vi "Motor and Two Photon System_Main.vi"() -> ()   [LabVIEW 2016]
doc: "This Continuous Measurement sample project is based on the Queued Message Handler template.\n\nThe Event Handling Loop generates messages based on user interface actions.\n\nThe Message Handling Loop processes messages generated by the Event Handling Loop, or by other messages. There are also Acquisition and Logging message handling loop subVIs, and a chart updating loop."
uses:
  Settings/Settings.ctl
  Acquisition/Hardware Configuration.ctl
  Logging/Logging Configuration.ctl
  Motor Speed/MSpeed AO HW Config.ctl
  Motor Control/Motor Control Config.ctl
  Motor Control/Speed and Duration.ctl
  2P Trigger/2P Trigger Config.ctl
  controls/UI Data.ctl
  controls/UI State.ctl
  support/Message Queue/Enqueue Message (Single).vi
  <vilib>/Utility/error.llb/Error Cluster From Error Code.vi
  <vilib>/ErrorRing/Error Ring.xnode
  Acquisition/Acquisition.lvlib
  Logging/Logging.lvlib
  Settings/Settings.lvlib
  support/User Event - Stop/User Event - Stop.lvlib
  support/Message Queue/Message Queue.lvlib
  Motor Speed/Motor Speed AO.lvlib
  Motor Control/Motor Control.lvlib
  2P Trigger/2P Trigger.lvlib
panel:
  out "Data":waveform(dbl)[](graph)
  in  "Force Trigger":bool
  in  "Settings":bool
  in  "Start":bool
  in  "Stop":bool
  out "Status":string
  in  "Exit":bool
  # "Continuous Measurement and Logging (NI-DAQmx)"
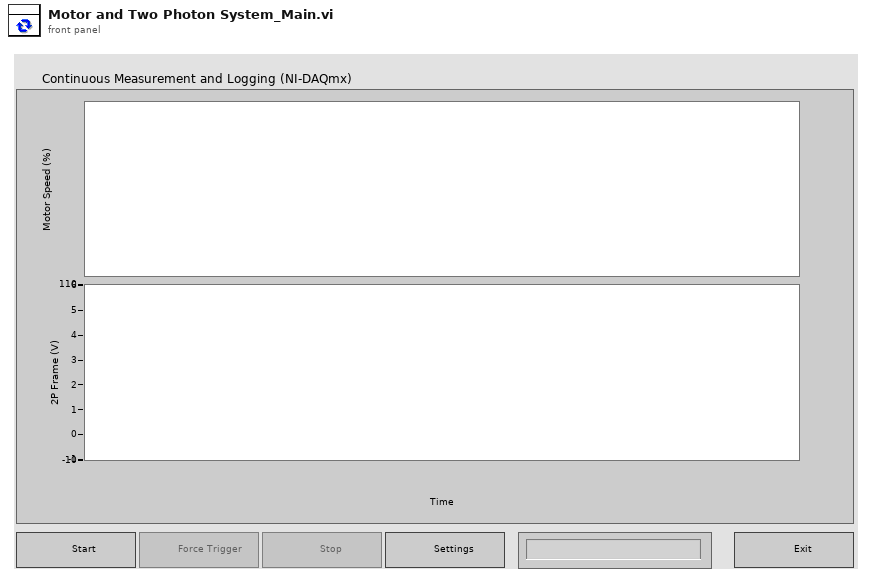
[diagram p1: front panel]
types:
  T1 = typedef "UI State.ctl" = enum16{"Idle", "Acquiring and Logging", "Waiting for Exit", "Waiting for Exit (Acq Stopped)", "Waiting for Exit (Log Stopped)", "Waiting for Stop", "Waiting for Stop (Acq Stopped)", "Waiting for Stop (Log Stopped)"}
  T2 = typedef "UI Data.ctl" = cluster{"Start Ref":refnum<vi>, "Trigger Ref":refnum<vi>, "Stop Ref":refnum<vi>, "Settings Ref":refnum<vi>, "Status Ref":refnum<vi>, "Exit Ref":refnum<vi>, "Data Ref":refnum<vi>}
  T3 = typedef "Settings.lvlib/Settings.ctl" = cluster{"Hardware Configuration":T4, "Logging Configuration":T5, "MSpeed AO HW Config":T6, "Motor Config":T7, "2P Trigger Config":T9}
  T4 = typedef "Acquisition.lvlib/Hardware Configuration.ctl" = cluster{"DAQmx Channel":tag, "Max Input":dbl, "Min Input":dbl, "Sample Rate":dbl, "DAQmx Task":refnum<k21>}
  T5 = typedef "Logging.lvlib/Logging Configuration.ctl" = cluster{"Log File Base Path":path, "TDMS File Reference":refnum<k34>, "Samples to Save":u32, "Trigger - Time":u32, "Trigger - Threshold":dbl, "Trigger - Channel":u32, "Enable Time Trigger":bool, "Enable Threshold Trigger":bool, "Always Log":bool}
  T6 = typedef "Motor Speed AO.lvlib/MSpeed AO HW Config.ctl" = cluster{"MSpeed AO Channel":tag, "Sample Rate(Hz)":dbl, "MSpeed AO Task":refnum<k21>}
  T7 = typedef "Motor Control.lvlib/Motor Control Config.ctl" = cluster{"VISA resource name":refnum<visa-resource-name>, "Speed and Duration":T8[]}
  T8 = typedef "Motor Control.lvlib/Speed and Duration.ctl" = cluster{"Speed (%)":i32, "Duration (sec)":dbl}
  T9 = typedef "2P Trigger.lvlib/2P Trigger Config.ctl" = cluster{"DO Line":tag}
  T10 = typedef "Message Queue.lvlib/All Message Queues.ctl" = cluster{"UI":refnum<queue>, "Acquisition":refnum<queue>, "Logging":refnum<queue>, "Motor Speed":refnum<queue>, "Motor Control":refnum<queue>, "2P Trigger":refnum<queue>}
  T11 = enum8{"Enabled", "Disabled", "Disabled and Grayed Out"}
  T12 = cluster{"MSpeed AO HW Config":T6, "VISA resource name":refnum<visa-resource-name>}
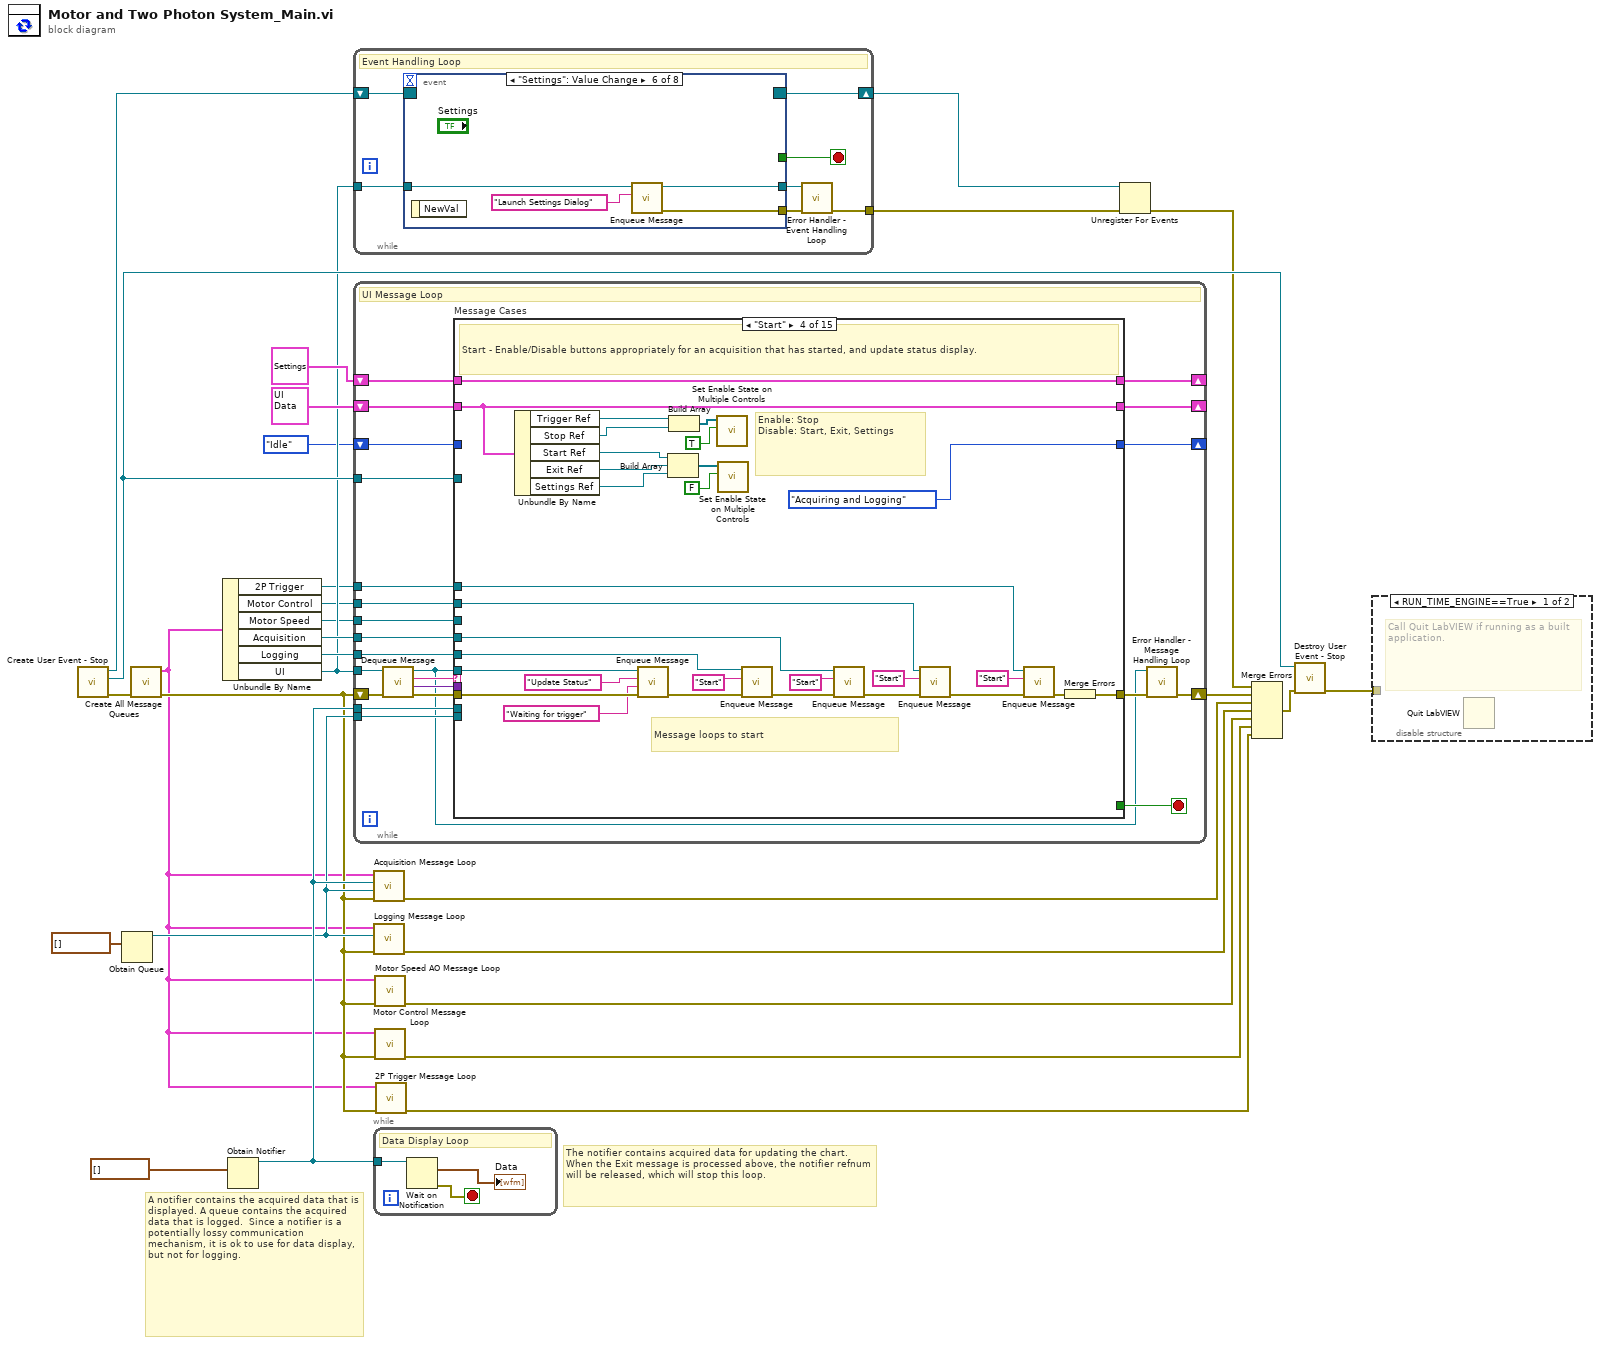
[diagram p0: block diagram]
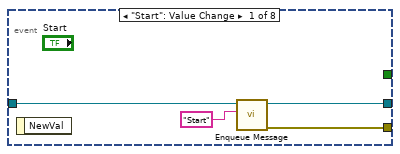
[diagram p3: hidden frame]
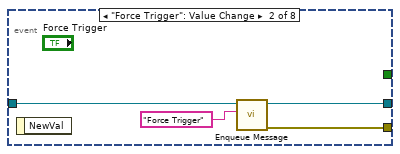
[diagram p4: hidden frame]
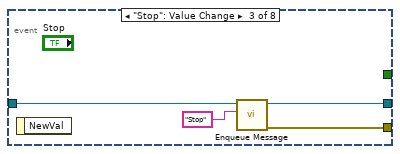
[diagram p5: hidden frame]
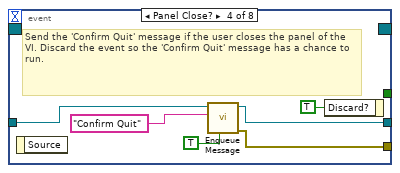
[diagram p6: hidden frame]
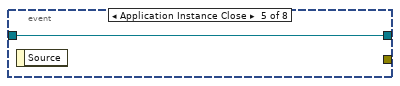
[diagram p7: hidden frame]
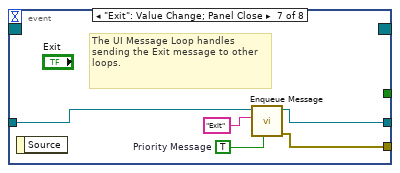
[diagram p8: hidden frame]
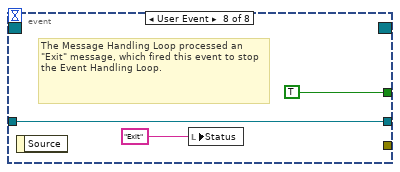
[diagram p9: hidden frame]
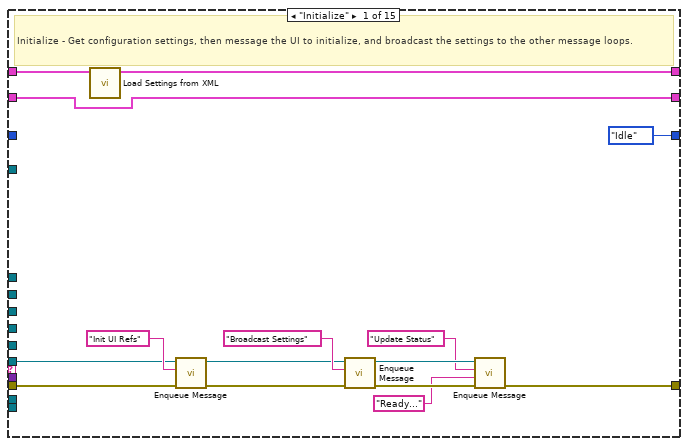
[diagram p10: hidden frame]
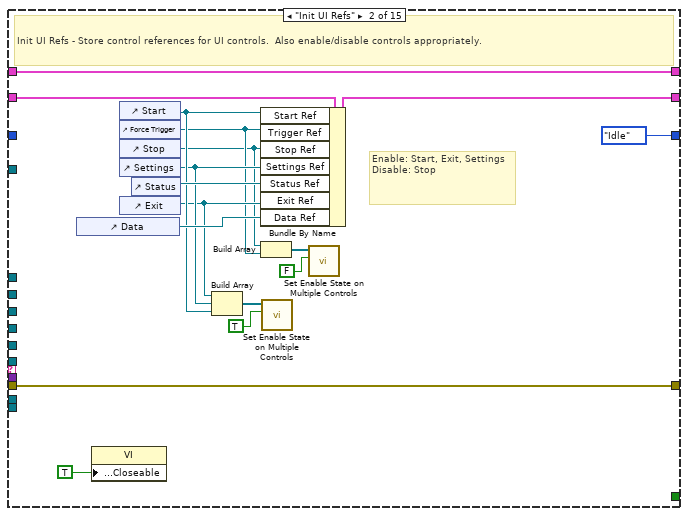
[diagram p11: hidden frame]
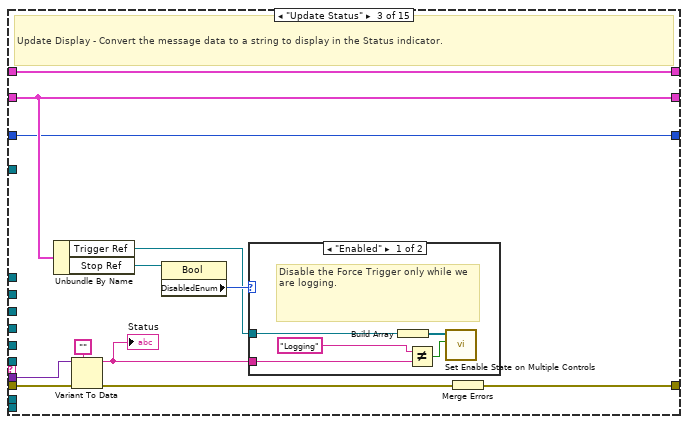
[diagram p12: hidden frame]
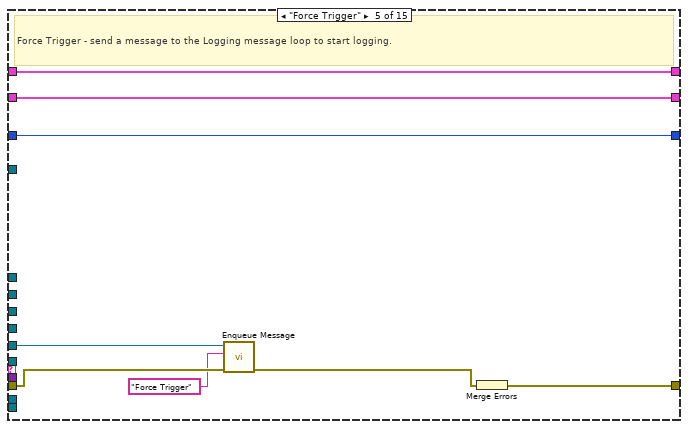
[diagram p14: hidden frame]
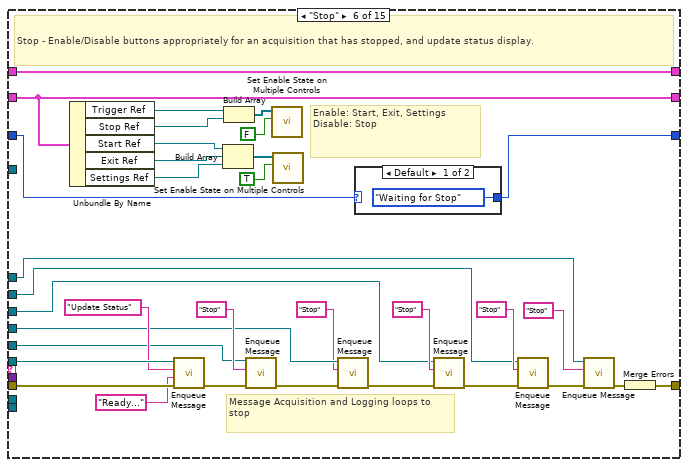
[diagram p15: hidden frame]
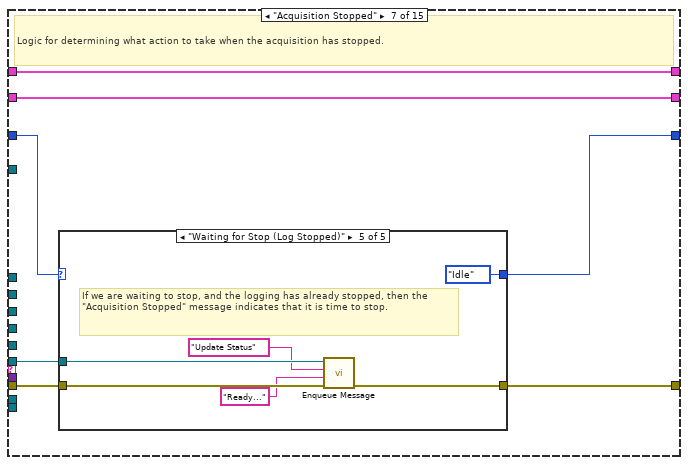
[diagram p17: hidden frame]
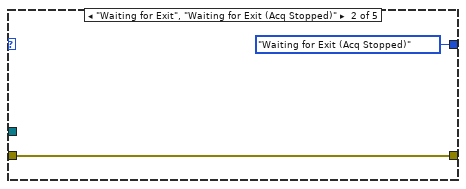
[diagram p19: hidden frame]
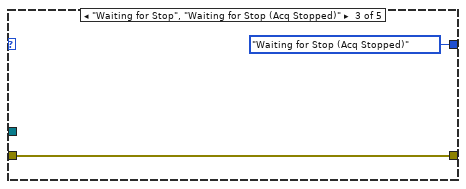
[diagram p20: hidden frame]
diagram:
  # "A notifier contains the acquired data that is displayed. A queue contains the acquired data that is logged.  Since a notifier is a potentially lossy communication mechanism, it is ok to use for data display, but not for logging."
  # "The notifier contains acquired data for updating the chart. When the Exit message is processed above, the notifier refnum will be released, which will stop this loop."
  n1 = call "Create User Event - Stop.vi"() -> ("error out"=w23:errorcluster, "User Event - Stop"=w25:refnum<user-event>, "Stop Event Registration Refnum"=w26:refnum<event-registration>)  [unwired: 9 in]
  n2 = Obtain Queue(element data type=waveform(dbl)[] []) -> (queue out=w6:refnum<queue>)  [unwired: 4 in, 2 out]
  n3 = call "Create All Message Queues.vi"("error in (no error)"=w23) -> ("error out"=w4:errorcluster, "Message Queues out"=w3:T10)  [unwired: 9 in]
  n4 = Unbundle By Name(w3) -> ("2P Trigger"=w1:refnum<queue>, "Motor Control"=w7:refnum<queue>, "Motor Speed"=w8:refnum<queue>, "Acquisition"=w17:refnum<queue>, "Logging"=w16:refnum<queue>, "UI"=w15:refnum<queue>)
  n5 = Obtain Notifier(notification data type=waveform(dbl)[] []) -> (notifier out=w13:refnum<notifier>)  [unwired: 3 in, 2 out]
  n6 = while {
    tunnel: w15 -> [w35]
    tunnel: [w30] -> w28
    shift-right: [w34] -> w19
    shift-left: w26 -> [w36]
    stop <- w33 stop-if-true
    # "Event Handling Loop"
    n7 = event shown="[5] \"Settings\": Value Change" {
      selector: w36 -> [_ _ _ _ _ _ _ _]
      dyn-events: [_ _ _ _ _ _ _ _] -> w34
      timeout: _ -> [_ _ _ _ _ _ _ _]
      tunnel: [_ _ _ _ _ _ _ TRUE ("Discard?")] -> w33
      tunnel: w35 -> [w38 w43 w47 w54 w55 w57 w61 w65]
      tunnel: [w40 w42 w46 w49 _ w59 w64 _] -> w31
      tunnel: [w37 w41 w45 w50 w55 w56 w60 w65] -> w32
      event "Start": Value Change {
        n8 = event-data() -> ()  [unwired: 1 in, 1 out]
        n9 = call-poly "Enqueue Message.vi"("Message"="Start", "Message Queue"=w38) -> ("error out"=w40:errorcluster, "dup Message Queue"=w37:refnum<queue>)  [unwired: 8 in]
      }
      event "Force Trigger": Value Change {
        n10 = event-data() -> ()  [unwired: 1 in, 1 out]
        n11 = call-poly "Enqueue Message.vi"("Message"="Force Trigger", "Message Queue"=w43) -> ("error out"=w42:errorcluster, "dup Message Queue"=w41:refnum<queue>)  [unwired: 8 in]
      }
      event "Stop": Value Change {
        n12 = event-data() -> ()  [unwired: 1 in, 1 out]
        n13 = call-poly "Enqueue Message.vi"("Message"="Stop", "Message Queue"=w47) -> ("error out"=w46:errorcluster, "dup Message Queue"=w45:refnum<queue>)  [unwired: 8 in]
      }
      event Panel Close? {
        # "Send the 'Confirm Quit' message if the user closes the panel of the VI. Discard the event so the 'Confirm Quit' message has a chance to run."
        n14 = event-data() -> ()  [unwired: 1 in, 1 out]
        n15 = call-poly "Enqueue Message.vi"("Priority Message? (F)"=TRUE, "Message"="Confirm Quit", "Message Queue"=w54) -> ("error out"=w49:errorcluster, "dup Message Queue"=w50:refnum<queue>)  [unwired: 7 in]
        n16 = event-data("Discard?"=TRUE) -> ()  [unwired: 1 in, 1 out]
      }
      event Application Instance Close {
        n17 = event-data() -> ()  [unwired: 1 in, 1 out]
      }
      event "Settings": Value Change {
        n18 = event-data() -> ()  [unwired: 1 in, 1 out]
        n19 = call-poly "Enqueue Message.vi"("Message"="Launch Settings Dialog", "Message Queue"=w57) -> ("error out"=w59:errorcluster, "dup Message Queue"=w56:refnum<queue>)  [unwired: 8 in]
      }
      event "Exit": Value Change; Panel Close {
        w62 = TRUE  # Priority Message
        # "The UI Message Loop handles sending the Exit message to other loops."
        n20 = event-data() -> ()  [unwired: 1 in, 1 out]
        n21 = call-poly "Enqueue Message.vi"("Priority Message? (F)"=w62, "Message"="Exit", "Message Queue"=w61) -> ("error out"=w64:errorcluster, "dup Message Queue"=w60:refnum<queue>)  [unwired: 7 in]
      }
      event User Event {
        # "The Message Handling Loop processed an \"Exit\" message, which fired this event to stop the Event Handling Loop."
        n22 = event-data() -> ()  [unwired: 1 in, 1 out]
        n23 = local write "Status"("Exit" ("Exit String")) -> ()
      }
    }
    n24 = call "Error Handler - Event Handling Loop.vi"("error in (no error)"=w31, "Message Queue"=w32) -> ("dup error in"=w30:errorcluster)  [unwired: 8 in, 1 out]
  }
  n25 = while {
    tunnel: w15 -> [w84]
    tunnel: w25 -> [w89]
    shift-right: [w74] -> w29
    shift-left: w4 -> [w88]
    shift-right: [w83] -> _
    shift-left: T3 {"Hardware Configuration"={"DAQmx Channel"="", "Max Input"=0.0, "Min Input"=0.0, "Sample Rate"=0.0, "DAQmx Task"=""}, "Logging Configuration"={"Log File Base Path"=path "", "TDMS File Reference"=refnum, "Samples to Save"=0, "Trigger - Time"=0, "Trigger - Threshold"=0.0, "Trigger - Channel"=0, "Enable Time Trigger"=FALSE, "Enable Threshold Trigger"=FALSE, "Always Log"=FALSE}, "MSpeed AO HW Config"={"MSpeed AO Channel"="", "Sample Rate(Hz)"=1000.0, "MSpeed AO Task"=""}, "Motor Config"={"VISA resource name"="", "Speed and Duration"=[{"Speed (%)"=10, "Duration (sec)"=120.0}, {"Speed (%)"=25, "Duration (sec)"=120.0}, {"Speed (%)"=50, "Duration (sec)"=120.0}]}, "2P Trigger Config"={"DO Line"="Dev1/port0/line0"}} ("Settings") -> [w82]
    shift-right: [w80] -> _
    shift-left: T2 {"Start Ref"=refnum, "Trigger Ref"=refnum, "Stop Ref"=refnum, "Settings Ref"=refnum, "Status Ref"=refnum, "Exit Ref"=refnum, "Data Ref"=refnum} ("Measurement UI Controls") -> [w81]
    tunnel: w17 -> [w79]
    tunnel: w16 -> [w78]
    tunnel: w13 -> [w77]
    tunnel: w6 -> [w76]
    shift-right: [w71] -> _
    shift-left: UI_State."Idle" ("UI State") -> [w72]
    tunnel: w8 -> [w70]
    tunnel: w7 -> [w69]
    tunnel: w1 -> [w68]
    stop <- w90 stop-if-true
    # "UI Message Loop"
    n26 = call "Dequeue Message.vi"("error in (no error)"=w88, "Message Queue"=w84) -> ("error out"=w87:errorcluster, "Message Data"=w85:variant, "Message"=w86:string, "dup Message Queue"=w73:refnum<queue>)  [unwired: 6 in]
    n27 = case "Message Cases" shown="\"Start\"" w86 {
      selector: w86 -> [_ _ _ _ _ _ _ _ _ _ _ _ _ _ w372]
      tunnel: w73 -> [w95 _ _ w167 _ w209 w213 w238 _ w291 w306 w316 w356 _ _]
      tunnel: w87 -> [w94 w122 w133 w166 w173 w208 w215 w240 w281 w293 w310 w315 w363 w370 _]
      tunnel: [w101 w122 w134 w168 w176 w210 w214 w239 w285 w288 w301 w314 w364 w369 w373] -> w75
      tunnel: [_ _ _ _ _ _ _ _ _ _ _ _ TRUE _ _] -> w90
      tunnel: w85 -> [_ _ w132 _ _ _ _ _ _ _ w309 _ _ _ _]
      tunnel: w89 -> [_ _ _ _ _ _ _ _ _ _ _ _ w362 _ _]
      tunnel: [w104 w121 w129 w165 w175 w207 w219 w244 w264 w290 w312 w319 w360 w368 w375] -> w83
      tunnel: w82 -> [w105 w121 w129 w165 w175 w207 w219 w244 w264 w294 w312 w319 w360 w368 w375]
      tunnel: w81 -> [w97 w120 w128 w162 w174 w204 w218 w243 w280 w287 w311 w318 w359 w367 w374]
      tunnel: [w97 w119 w128 w162 w174 w204 w218 w243 w280 w287 w311 w318 w359 w367 w374] -> w80
      tunnel: w79 -> [_ _ _ w150 _ w192 _ _ w279 _ _ _ w358 _ _]
      tunnel: w78 -> [_ _ _ w152 w170 w194 _ _ w278 _ _ _ w357 _ _]
      tunnel: w77 -> [_ _ _ _ _ _ _ _ _ _ _ _ w355 _ _]
      tunnel: w76 -> [_ _ _ _ _ _ _ _ _ _ _ _ w351 _ _]
      tunnel: w72 -> [_ _ w123 _ w169 w188 w217 w242 w277 w286 w300 w317 _ w366 w371]
      tunnel: [UI_State."Idle" ("UI State") UI_State."Idle" ("UI State") w123 UI_State."Acquiring and Logging" ("UI State") w169 w187 w216 w241 w277 w286 w300 w313 UI_State."Idle" ("UI State") w366 w371] -> w71
      tunnel: w70 -> [_ _ _ _ _ w184 _ _ w275 _ _ _ w346 _ _]
      tunnel: w69 -> [_ _ _ w143 _ w181 _ _ w273 _ _ _ w344 _ _]
      tunnel: w68 -> [_ _ _ w140 _ w178 _ _ w265 _ _ _ w341 _ _]
      frame "Initialize" {
        # "Initialize - Get configuration settings, then message the UI to initialize, and broadcast the settings to the other message loops."
        n28 = call "Load Settings from XML.vi"("Settings in"=w105) -> ("Settings out"=w104:T3)  [unwired: 9 in, 1 out]
        n29 = call-poly "Enqueue Message.vi"("error in (no error)"=w94, "Message"="Init UI Refs", "Message Queue"=w95) -> ("error out"=w92:errorcluster, "dup Message Queue"=w93:refnum<queue>)  [unwired: 7 in]
        n30 = call-poly "Enqueue Message.vi"("error in (no error)"=w92, "Message"="Broadcast Settings", "Message Queue"=w93) -> ("error out"=w103:errorcluster, "dup Message Queue"=w102:refnum<queue>)  [unwired: 7 in]
        n31 = call-poly "Enqueue Message.vi"("error in (no error)"=w103, "Message Data"="Ready..." ("Ready..."), "Message"="Update Status", "Message Queue"=w102) -> ("error out"=w101:errorcluster)  [unwired: 6 in, 1 out]
      }
      frame "Init UI Refs" {
        # "Enable: Start, Exit, Settings\nDisable: Stop"
        # "Init UI Refs - Store control references for UI controls.  Also enable/disable controls appropriately."
        n32 = control-ref of="Data"() -> (w115:refnum<vi>)
        n33 = property class="VI"("Front Panel.Closeable"=TRUE ("Front Panel Window:Closeable")) -> ()  [unwired: 2 in, 2 out]
        n34 = control-ref of="Start"() -> (w114:refnum<vi>)
        n35 = control-ref of="Force Trigger"() -> (w109:refnum<vi>)
        n36 = control-ref of="Stop"() -> (w108:refnum<vi>)
        n37 = control-ref of="Settings"() -> (w111:refnum<vi>)
        n38 = control-ref of="Exit"() -> (w110:refnum<vi>)
        n39 = control-ref of="Status"() -> (w116:refnum<vi>)
        n40 = Build Array(w110, w111, w114) -> (w113:refnum<vi>[])
        n41 = Bundle By Name(cluster=w120, "Start Ref"=w114, "Trigger Ref"=w109, "Stop Ref"=w108, "Settings Ref"=w111, "Status Ref"=w116, "Exit Ref"=w110, "Data Ref"=w115) -> (w119:T2)
        n42 = Build Array(w108, w109) -> (w107:refnum<vi>[])
        n43 = call "Set Enable State on Multiple Controls.vi"("Enable?"=TRUE, "Controls"=w113) -> ()  [unwired: 10 in]
        n44 = call "Set Enable State on Multiple Controls.vi"("Enable?"=FALSE, "Controls"=w107) -> ()  [unwired: 10 in]
      }
      frame "Update Status" {
        # "Update Display - Convert the message data to a string to display in the Status indicator."
        n45 = Unbundle By Name(w128) -> ("Trigger Ref"=w124:refnum<vi>, "Stop Ref"=w127:refnum<vi>)
        n46 = Variant To Data(error in=w133, type="", Variant=w132) -> (data=w125:string, error out=w130:errorcluster)
        "Status" <- w125
        n47 = property class="Bool"(reference=w127) -> ("DisabledEnum"=w126:T11)  [unwired: 1 in, 2 out]
        n48 = case shown="\"Enabled\"" w126 {
          tunnel: w125 -> [w137 _]
          tunnel: w124 -> [w138 _]
          frame "Enabled" {
            # "Disable the Force Trigger only while we are logging."
            n49 = Build Array(w138) -> (w139:refnum<vi>[])
            n50 = Not Equal?(x="Logging" ("Logging"), y=w137) -> (x != y?=w135:bool)
            n51 = call "Set Enable State on Multiple Controls.vi"("Enable?"=w135, "Controls"=w139) -> ()  [unwired: 10 in]
          }
          frame "Disabled", Default {
          }
        }
        n52 = Merge Errors(w130) -> (w134:errorcluster)
      }
      frame "Start" {
        # "Message loops to start"
        # "Enable: Stop\nDisable: Start, Exit, Settings"
        # "Start - Enable/Disable buttons appropriately for an acquisition that has started, and update status display."
        n53 = Unbundle By Name(w162) -> ("Trigger Ref"=w147:refnum<vi>, "Stop Ref"=w148:refnum<vi>, "Start Ref"=w157:refnum<vi>, "Exit Ref"=w156:refnum<vi>, "Settings Ref"=w155:refnum<vi>)
        n54 = call-poly "Enqueue Message.vi"("error in (no error)"=w166, "Message Data"="Waiting for trigger" ("Waiting for trigger"), "Message"="Update Status", "Message Queue"=w167) -> ("error out"=w154:errorcluster)  [unwired: 6 in, 1 out]
        n55 = Build Array(w157, w156, w155) -> (w160:refnum<vi>[])
        n56 = Build Array(w147, w148) -> (w159:refnum<vi>[])
        n57 = call "Set Enable State on Multiple Controls.vi"("Enable?"=TRUE, "Controls"=w159) -> ()  [unwired: 10 in]
        n58 = call "Set Enable State on Multiple Controls.vi"("Enable?"=FALSE, "Controls"=w160) -> ()  [unwired: 10 in]
        n59 = call-poly "Enqueue Message.vi"("error in (no error)"=w154, "Message"="Start", "Message Queue"=w152) -> ("error out"=w151:errorcluster)  [unwired: 7 in, 1 out]
        n60 = call-poly "Enqueue Message.vi"("error in (no error)"=w151, "Message"="Start", "Message Queue"=w150) -> ("error out"=w142:errorcluster)  [unwired: 7 in, 1 out]
        n61 = call-poly "Enqueue Message.vi"("error in (no error)"=w142, "Message"="Start", "Message Queue"=w143) -> ("error out"=w144:errorcluster)  [unwired: 7 in, 1 out]
        n62 = call-poly "Enqueue Message.vi"("Message"="Start", "Message Queue"=w140) -> ()  [unwired: 8 in, 2 out]
        n63 = Merge Errors(w144) -> (w168:errorcluster)
      }
      frame "Force Trigger" {
        # "Force Trigger - send a message to the Logging message loop to start logging."
        n64 = call-poly "Enqueue Message.vi"("error in (no error)"=w173, "Message"="Force Trigger", "Message Queue"=w170) -> ("error out"=w172:errorcluster)  [unwired: 7 in, 1 out]
        n65 = Merge Errors(w172) -> (w176:errorcluster)
      }
      frame "Stop" {
        # "Message Acquisition and Logging loops to stop"
        # "Enable: Start, Exit, Settings\nDisable: Stop"
        # "Stop - Enable/Disable buttons appropriately for an acquisition that has stopped, and update status display."
        n66 = Unbundle By Name(w204) -> ("Trigger Ref"=w189:refnum<vi>, "Stop Ref"=w190:refnum<vi>, "Start Ref"=w199:refnum<vi>, "Exit Ref"=w198:refnum<vi>, "Settings Ref"=w197:refnum<vi>)
        n67 = call-poly "Enqueue Message.vi"("error in (no error)"=w208, "Message Data"="Ready..." ("Ready..."), "Message"="Update Status", "Message Queue"=w209) -> ("error out"=w196:errorcluster)  [unwired: 6 in, 1 out]
        n68 = Build Array(w199, w198, w197) -> (w202:refnum<vi>[])
        n69 = Build Array(w189, w190) -> (w201:refnum<vi>[])
        n70 = call-poly "Enqueue Message.vi"("error in (no error)"=w196, "Message"="Stop", "Message Queue"=w194) -> ("error out"=w193:errorcluster)  [unwired: 7 in, 1 out]
        n71 = call "Set Enable State on Multiple Controls.vi"("Enable?"=FALSE, "Controls"=w201) -> ()  [unwired: 10 in]
        n72 = call "Set Enable State on Multiple Controls.vi"("Enable?"=TRUE, "Controls"=w202) -> ()  [unwired: 10 in]
        n73 = call-poly "Enqueue Message.vi"("error in (no error)"=w193, "Message"="Stop", "Message Queue"=w192) -> ("error out"=w185:errorcluster)  [unwired: 7 in, 1 out]
        n74 = case shown="Default" w188 {
          selector: w188 -> [_ w212]
          tunnel: [UI_State."Waiting for Stop" ("UI State") w212] -> w187
          frame Default {
          }
          frame "Waiting for Exit" {
          }
        }
        n75 = call-poly "Enqueue Message.vi"("error in (no error)"=w185, "Message"="Stop", "Message Queue"=w184) -> ("error out"=w182:errorcluster)  [unwired: 7 in, 1 out]
        n76 = call-poly "Enqueue Message.vi"("error in (no error)"=w182, "Message"="Stop", "Message Queue"=w181) -> ("error out"=w180:errorcluster)  [unwired: 7 in, 1 out]
        n77 = call-poly "Enqueue Message.vi"("error in (no error)"=w180, "Message"="Stop", "Message Queue"=w178) -> ("error out"=w179:errorcluster)  [unwired: 7 in, 1 out]
        n78 = Merge Errors(w179) -> (w210:errorcluster)
      }
      frame "Acquisition Stopped" {
        # "Logic for determining what action to take when the acquisition has stopped."
        n79 = case shown="\"Waiting for Stop (Log Stopped)\"" w217 {
          selector: w217 -> [w221 _ _ _ _]
          tunnel: [w221 UI_State."Waiting for Exit (Acq Stopped)" ("UI State") UI_State."Waiting for Stop (Acq Stopped)" ("UI State") UI_State."Idle" ("UI State") UI_State."Idle" ("UI State")] -> w216
          tunnel: w215 -> [w220 w222 w224 w230 w236]
          tunnel: [w220 w222 w224 w229 w235] -> w214
          tunnel: w213 -> [_ _ _ w228 w234]
          frame Default {
          }
          frame "Waiting for Exit", "Waiting for Exit (Acq Stopped)" {
          }
          frame "Waiting for Stop", "Waiting for Stop (Acq Stopped)" {
          }
          frame "Waiting for Exit (Log Stopped)" {
            # "If we are waiting to exit, and the logging has already stopped, then the \"Acquisition Stopped\" message indicates that it is time to exit."
            n80 = call-poly "Enqueue Message.vi"("Priority Message? (F)"=TRUE, "error in (no error)"=w230, "Message"="Exit", "Message Queue"=w228) -> ("error out"=w229:errorcluster)  [unwired: 6 in, 1 out]
          }
          frame "Waiting for Stop (Log Stopped)" {
            # "If we are waiting to stop, and the logging has already stopped, then the \"Acquisition Stopped\" message indicates that it is time to stop."
            n81 = call-poly "Enqueue Message.vi"("error in (no error)"=w236, "Message Data"="Ready..." ("Message"), "Message"="Update Status", "Message Queue"=w234) -> ("error out"=w235:errorcluster)  [unwired: 6 in, 1 out]
          }
        }
      }
      frame "Logging Stopped" {
        # "Logic for determining what action to take when the logging has stopped."
        n82 = case shown="\"Waiting for Stop (Acq Stopped)\"" w242 {
          selector: w242 -> [w246 _ _ _ _]
          tunnel: [w246 UI_State."Waiting for Exit (Log Stopped)" ("UI State") UI_State."Waiting for Stop (Log Stopped)" ("UI State") UI_State."Idle" ("UI State") UI_State."Idle" ("UI State")] -> w241
          tunnel: w240 -> [w245 w247 w249 w255 w261]
          tunnel: [w245 w247 w249 w254 w260] -> w239
          tunnel: w238 -> [_ _ _ w253 w259]
          frame Default {
          }
          frame "Waiting for Exit", "Waiting for Exit (Log Stopped)" {
          }
          frame "Waiting for Stop", "Waiting for Stop (Log Stopped)" {
          }
          frame "Waiting for Exit (Acq Stopped)" {
            # "If we are waiting to exit, and the acquisition has already stopped, then the \"Logging Stopped\" message indicates that it is time to exit."
            n83 = call-poly "Enqueue Message.vi"("Priority Message? (F)"=TRUE, "error in (no error)"=w255, "Message"="Exit", "Message Queue"=w253) -> ("error out"=w254:errorcluster)  [unwired: 6 in, 1 out]
          }
          frame "Waiting for Stop (Acq Stopped)" {
            # "If we are waiting to stop, and the acquisition has already stopped, then the \"Logging Stopped\" message indicates that it is time to stop."
            n84 = call-poly "Enqueue Message.vi"("error in (no error)"=w261, "Message Data"="Ready..." ("Message"), "Message"="Update Status", "Message Queue"=w259) -> ("error out"=w260:errorcluster)  [unwired: 6 in, 1 out]
          }
        }
      }
      frame "Broadcast settings" {
        w266 = "Update Settings" ("Message")
        # "Send the 'Update Settings' message to the Logging and Acquisition message loops."
        n85 = Unbundle By Name(w264) -> ("Hardware Configuration"=w283:T4, "Logging Configuration"=w282:T5)
        n86 = Unbundle By Name(w264) -> ("2P Trigger Config"=w263:T9)
        n87 = Unbundle By Name(w264) -> ("Motor Config"=w272:T7, "MSpeed AO HW Config"=w270:T6, "Motor Config.VISA resource name"=w271:refnum<visa-resource-name>)
        n88 = call-poly "Enqueue Message.vi"("Message Data"=w283, "Message"=w266, "Message Queue"=w279) -> ("error out"=w284:errorcluster)  [unwired: 7 in, 1 out]
        n89 = Bundle("MSpeed AO HW Config"=w270, "VISA resource name"=w271) -> (w269:T12)  [unwired: 1 in]
        n90 = call-poly "Enqueue Message.vi"("error in (no error)"=w284, "Message Data"=w282, "Message"=w266, "Message Queue"=w278) -> ("error out"=w276:errorcluster)  [unwired: 6 in, 1 out]
        n91 = call-poly "Enqueue Message.vi"("error in (no error)"=w276, "Message Data"=w269, "Message"=w266, "Message Queue"=w275) -> ("error out"=w274:errorcluster)  [unwired: 6 in, 1 out]
        n92 = call-poly "Enqueue Message.vi"("error in (no error)"=w274, "Message Data"=w272, "Message"=w266, "Message Queue"=w273) -> ("error out"=w268:errorcluster)  [unwired: 6 in, 1 out]
        n93 = call-poly "Enqueue Message.vi"("error in (no error)"=w268, "Message Data"=w263, "Message"=w266, "Message Queue"=w265) -> ("error out"=w267:errorcluster)  [unwired: 6 in, 1 out]
        n94 = Merge Errors(w267, w281) -> (w285:errorcluster)
      }
      frame "Launch Settings Dialog" {
        # "Launch the Settings Dialog when the user clicks the 'Settings' button."
        n95 = call "Settings Dialog.vi"("error in (no error)"=w293, "Settings in"=w294) -> ("error out"=w289:errorcluster, "Cancelled?"=w292:bool, "Settings out"=w290:T3)  [unwired: 6 in, 1 out]
        n96 = case shown="False" w292 {
          tunnel: w291 -> [w298 _]
          tunnel: w289 -> [w297 w299]
          tunnel: [w296 w299] -> w288
          frame False {
            n97 = call-poly "Enqueue Message.vi"("error in (no error)"=w297, "Message"="Broadcast Settings", "Message Queue"=w298) -> ("error out"=w296:errorcluster)  [unwired: 7 in, 1 out]
          }
          frame True {
          }
        }
      }
      frame "Error" {
        # "Error - Check the error message data and respond accordingly. This message is sent by the \"Error Handler\" VIs at the end of each loop in this application."
        n98 = Variant To Data(error in=w310, type=errorcluster {"status"=FALSE, "code"=0, "source"=""} ("error out"), Variant=w309) -> (data=w307:errorcluster, error out=w303:errorcluster)
        n99 = call <vilib>:"Simple Error Handler.vi"("error in (no error)"=w307) -> ()  [unwired: 4 in, 5 out]
        n100 = call-poly "Enqueue Message.vi"("Priority Message? (F)"=TRUE, "Message"="Exit", "Message Queue"=w306) -> ("error out"=w302:errorcluster)  [unwired: 7 in, 1 out]
        n101 = Merge Errors(w302, w303) -> (w301:errorcluster)
      }
      frame "Confirm Quit" {
        # "Confirm Quit - Message that can confirm whether or not the user wants to exit the application."
        n102 = case shown="\"Acquiring and Logging\"" w317 {
          tunnel: w316 -> [w324 w330]
          tunnel: w315 -> [w323 w328]
          tunnel: [w320 w327] -> w314
          tunnel: [UI_State."Idle" ("UI State") w326] -> w313
          frame Default {
            # "If 'Confirm Quit' comes in while the system is idle, there is no need for a confirmation message."
            n103 = call-poly "Enqueue Message.vi"("Priority Message? (F)"=TRUE, "error in (no error)"=w323, "Message"="Exit", "Message Queue"=w324) -> ("error out"=w320:errorcluster)  [unwired: 6 in, 1 out]
          }
          frame "Acquiring and Logging" {
            n104 = Two Button Dialog(message="Are you sure you want to quit while the acquisition is running?" ("Confirm Quit Message"), 1:"No" ("No"), 2:"Yes" ("Yes")) -> (T button?=w329:bool)
            n105 = case shown="True" w329 {
              tunnel: w330 -> [_ w340]
              tunnel: w328 -> [w334 w339]
              tunnel: [w334 w338] -> w327
              tunnel: [UI_State."Acquiring and Logging" ("UI State") UI_State."Waiting for Exit" ("UI State")] -> w326
              frame False {
                # "User did not want to quit."
              }
              frame True {
                n106 = call-poly "Enqueue Message.vi"("error in (no error)"=w339, "Message"="Stop", "Message Queue"=w340) -> ("error out"=w338:errorcluster)  [unwired: 7 in, 1 out]
              }
            }
          }
        }
      }
      frame "Exit" {
        w342 = "Exit" ("Message")
        # "Don't check the error outs. The acquisition and logging queues may have already been released."
        # "Close references owned by the Main VI."
        # "Stop the VI"
        # "Exit - Fire the User Event to stop the Event Handling Loop.  Also send Exit messages to the Acquisition and Logging loops."
        n107 = Release Queue(queue=w356, error in (no error)=w363) -> (error out=w354:errorcluster)  [unwired: 1 in, 2 out]
        n108 = call "Fire User Event - Stop.vi"("User Event - Stop"=w362) -> ("error out"=w361:errorcluster)  [unwired: 10 in]
        n109 = Release Notifier(notifier=w355, error in (no error)=w354) -> (error out=w353:errorcluster)  [unwired: 1 in, 2 out]
        n110 = Release Queue(queue=w351, error in (no error)=w353) -> (error out=w352:errorcluster)  [unwired: 1 in, 2 out]
        n111 = call-poly "Enqueue Message.vi"("Priority Message? (F)"=TRUE, "Message"=w342, "Message Queue"=w358) -> ()  [unwired: 7 in, 2 out]
        n112 = call-poly "Enqueue Message.vi"("Priority Message? (F)"=TRUE, "Message"=w342, "Message Queue"=w357) -> ()  [unwired: 7 in, 2 out]
        n113 = call-poly "Enqueue Message.vi"("Priority Message? (F)"=TRUE, "Message"=w342, "Message Queue"=w346) -> ()  [unwired: 7 in, 2 out]
        n114 = call-poly "Enqueue Message.vi"("Priority Message? (F)"=TRUE, "Message"=w342, "Message Queue"=w344) -> ()  [unwired: 7 in, 2 out]
        n115 = call-poly "Enqueue Message.vi"("Priority Message? (F)"=TRUE, "Message"=w342, "Message Queue"=w341) -> ()  [unwired: 7 in, 2 out]
        n116 = Merge Errors(w361, w352) -> (w364:errorcluster)
      }
      frame "---Copy This Frame---" {
        # "Duplicate this frame when creating new messages.  Change this comment in the duplicated frame to describe this message."
        n117 = Merge Errors(w370) -> (w369:errorcluster)
      }
      frame Default {
        # "'Default' case only runs if there is a message that isn't defined in any of the other cases.  Output a programming error."
        n118 = xnode "Error Ring"("parameter 0"=w372) -> ("error out"=w373:errorcluster)
      }
    }
    n119 = call "Error Handler - Message Handling Loop.vi"("error in (no error)"=w75, "Message Queue"=w73) -> ("dup error in"=w74:errorcluster)  [unwired: 8 in, 1 out]
  }
  n120 = call "Acquisition Message Loop.vi"("error in (no error)"=w4, "Data Queue"=w6, "Data Notifier"=w13, "Message Queues"=w3) -> ("error out"=w24:errorcluster)  [unwired: 7 in]
  n121 = call "Logging Message Loop.vi"("error in (no error)"=w4, "Data Queue"=w6, "Message Queues"=w3) -> ("error out"=w22:errorcluster)  [unwired: 8 in]
  n122 = while "Data Display Loop" {
    tunnel: w13 -> [w385]
    stop <- w383 stop-if-true
    # "Data Display Loop"
    n123 = Wait on Notification(notifier=w385) -> (notification=→"Data":waveform(dbl)[], error out=w383:errorcluster)  [unwired: 3 in, 2 out]
  }
  n124 = call "Motor Speed AO Message Loop.vi"("error in (no error)"=w4, "Message Queues"=w3) -> ("error out"=w9:errorcluster)  [unwired: 9 in]
  n125 = call "Motor Control Message Loop.vi"("error in (no error)"=w4, "Message Queues"=w3) -> ("error out"=w5:errorcluster)  [unwired: 9 in]
  n126 = call "2P Trigger Message Loop.vi"("error in (no error)"=w4, "Message Queues"=w3) -> ("error out"=w2:errorcluster)  [unwired: 9 in]
  n127 = Unregister For Events(event registration refnum=w19, error in=w28) -> (error out=w20:errorcluster)
  n128 = Merge Errors(w20, w29, w24, w22, w9, w5, w2) -> (w27:errorcluster)
  n129 = call "Destroy User Event - Stop.vi"("error in (no error)"=w27, "User Event - Stop"=w25) -> ("error out"=w11:errorcluster)  [unwired: 9 in]
  n130 = disable-structure shown="RUN_TIME_ENGINE==True" {
    disable-tunnel: w11 -> [_ _]
    frame condition #0 {
      # "Call Quit LabVIEW if running as a built application."
      n131 = Quit LabVIEW() -> ()  [unwired: 1 in]
    }
    frame condition #1 (active) {
    }
  }
